vi "set_http_configuration.vi"(8 "error in (no error)":errorcluster, 11 "configuration":T1) -> (0 "error out":errorcluster)   [LabVIEW 2015, in "lv-dropbox.lvlib"]
uses:
  lv-dropbox.lvlib
  private/_controls/http_configuration.ctl
  private/_controls/fg_command.ctl
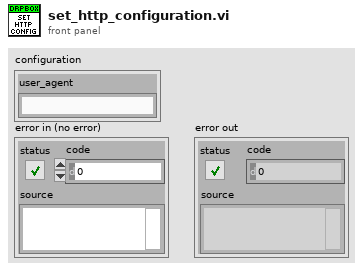
[diagram p1: front panel]
types:
  T1 = typedef "lv-dropbox.lvlib/http_configuration.ctl" = cluster{"user_agent":string}
  T2 = typedef "lv-dropbox.lvlib/fg_command.ctl" = enum16{"<fg_command>", "initialize", "read", "write", "shutdown"}
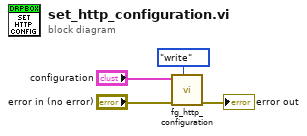
[diagram p0: block diagram]
diagram:
  n1 = call "fg_http_configuration.vi"("fg_command"=fg_command."write", "error in (no error)"="error in (no error)", "http_configuration in"="configuration") -> ("error out"=→"error out":errorcluster)  [unwired: 7 in, 1 out]
